vi "SaveArray.vi"(9 "data":dbl[][](array[numeric]), 11 "file path":path) -> ()   [LabVIEW 2010, in "KevLib01.lvlib"]
uses:
  KevLib01.lvlib
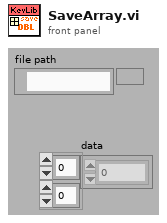
[diagram p1: front panel]
types:
  T1 = enum16{"open", "replace", "create", "open or create", "replace or create", "replace or create with confirmation"}
  T2 = enum16{"deny read/write", "deny write-only", "deny none"}
  T3 = enum16{"big-endian, network order", "native, host order", "little-endian"}
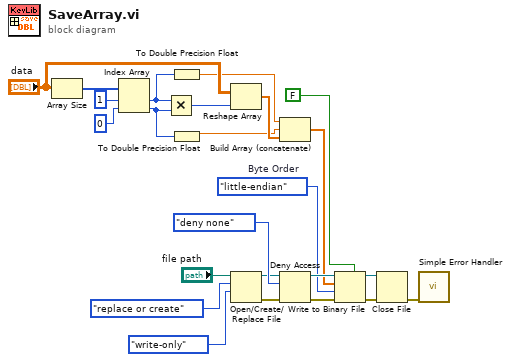
[diagram p0: block diagram]
diagram:
  w6 = T3."little-endian"  # Byte Order
  n1 = Array Size(array="data") -> (size(s)=w14:i32[])
  n2 = Index Array(array=w14, index #1=1 ("index"), index #2=0 ("index")) -> (element #1=w12:i32, element #2=w11:i32)
  n3 = Multiply(x=w12, y=w11) -> (x*y=w13:i32)
  n4 = To Double Precision Float(number=w12) -> (double precision float=w9:dbl)
  n5 = To Double Precision Float(number=w11) -> (double precision float=w8:dbl)
  n6 = Reshape Array("data", w13) -> (w10:dbl[])
  n7 = Open/Create/Replace File(file path (use dialog)="file path", operation (0:open)=T1."replace or create", access (0:read/write)=enum16{"read/write", "read-only", "write-only"}."write-only") -> (refnum out=w21:refnum<file>, error out=w20:errorcluster)  [unwired: 1 in, 3 out]
  n8 = Build Array (concatenate)(w9, w8, w10) -> (w7:dbl[])
  n9 = Deny Access(4:w20, 6:T2."deny none" ("deny mode (0:deny read/write)"), 7:w21) -> (0:w5:errorcluster, 3:w18:refnum<file>)
  n10 = Write to Binary File(file (use dialog)=w18, data=w7, error in=w5, 5:FALSE ("prepend array or string size? (T)"), 9:w6) -> (refnum out=w3:refnum<file>, error out=w2:errorcluster)  [unwired: 2 out]
  n11 = Close File(refnum=w3, error in=w2) -> (error out=w4:errorcluster)  [unwired: 1 out]
  n12 = call <vilib>:"Simple Error Handler.vi"("error in (no error)"=w4) -> ()  [unwired: 1 in, 8 out]
